vi "K2182A_Manage_Monitor.vi"(4 "System Monitor Variables (in)":T3, 5 "K2182A Cluster":T1 caption="Command (in)", 6 "Global Status (in)":T1, 7 "queue (in)":refnum<queue>) -> (0 "System Monitor Variables (out)":T3, 1 "Monitor (out)":T1)   [LabVIEW 2019]
uses:
  Global/Global Variables/System Monitor Cluster.ctl
  K2182A/K2812A_cluster.ctl
  Equipment/Keithley 622x/Configure/2182 -A/Low Level/Typedefs/KE2182 -- Voltage Ranges.ctl
  Equipment/Keithley 622x/Keithley 622x.lvlib
panel:
  # "K 2182A"
  # "K 2182A"
  # "K 2182A"
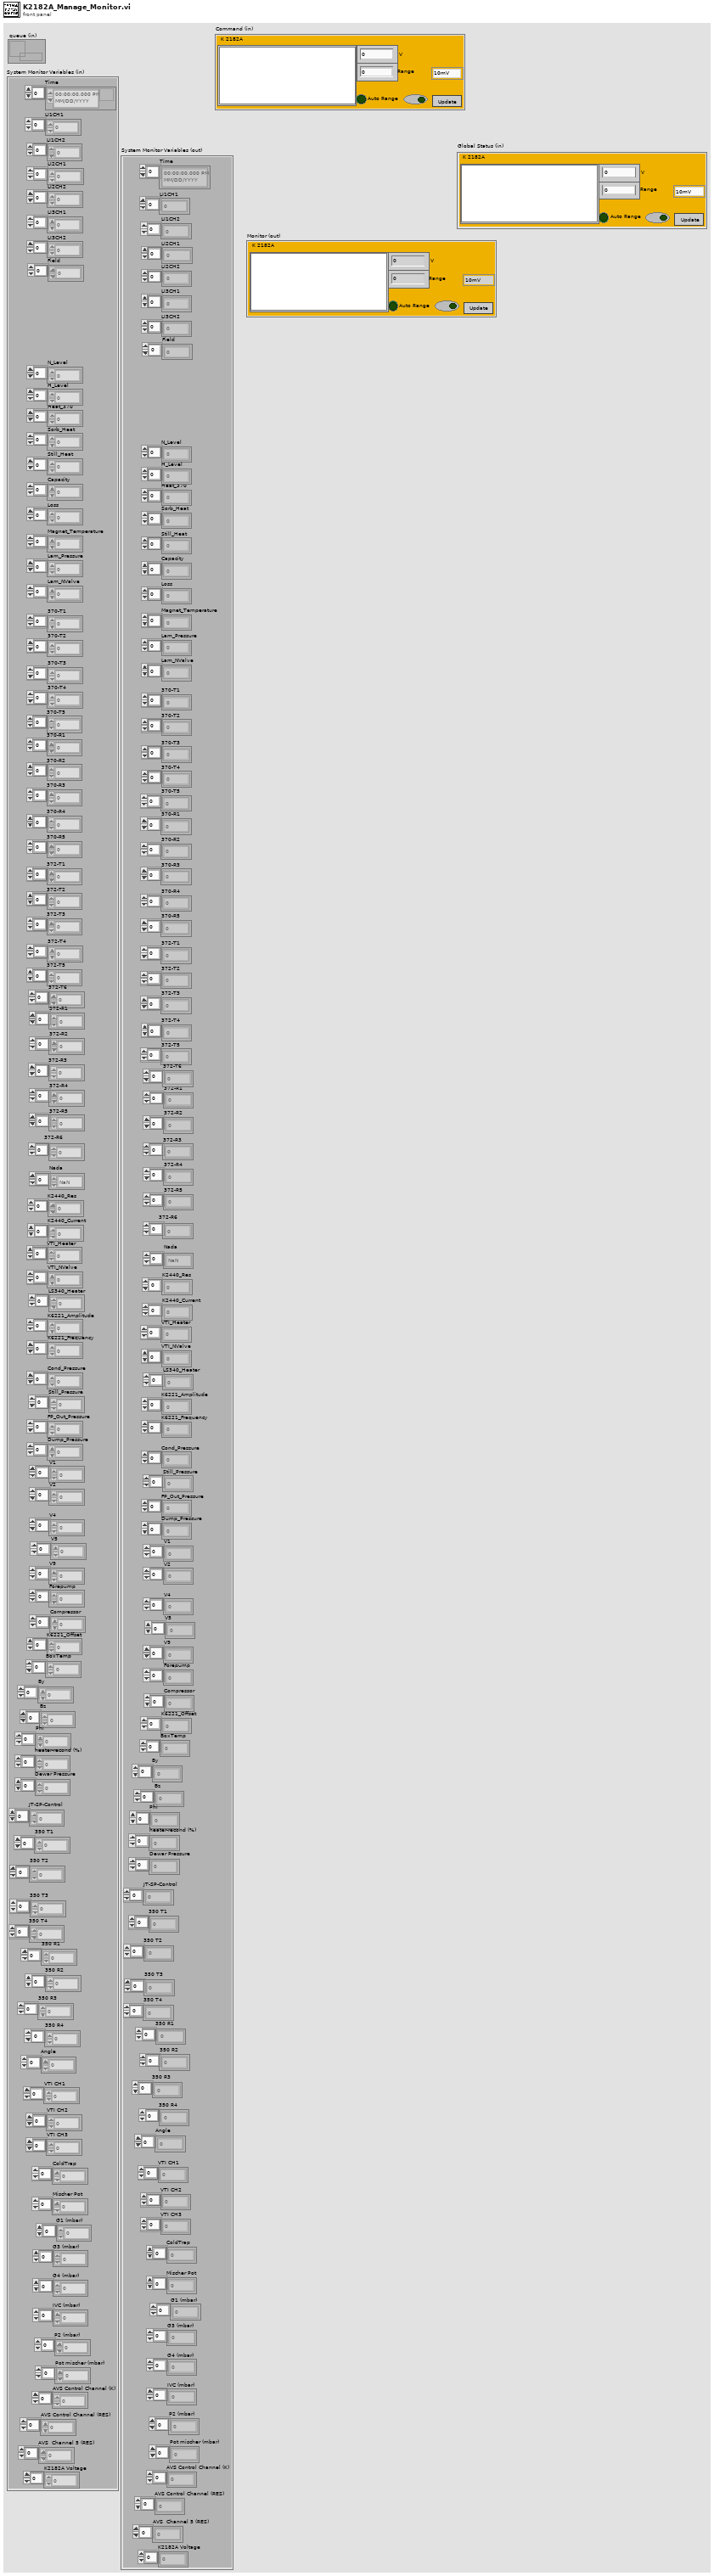
[diagram p1: front panel]
types:
  T1 = typedef "K2812A_cluster.ctl" = cluster{"Plot Window":dbl[][], "Range":dbl, "Update":bool, "Range selector":T2, "Auto Range":bool, "V":dbl, "Auto Range set":bool}
  T2 = typedef "Keithley 622x.lvlib/KE2182 -- Voltage Ranges.ctl" = enum16{"10mV", "100mV", "1V", "10V", "100V"}
  T3 = typedef "System Monitor Cluster.ctl" = cluster{"Time":timestamp[], "LI1CH1":dbl[], "LI1CH2":dbl[], "LI2CH1":dbl[], "LI2CH2":dbl[], "LI3CH1":dbl[], "LI3CH2":dbl[], "Field":dbl[], "N_Level":dbl[], "H_Level":dbl[], "Heat_370":dbl[], "Sorb_Heat":dbl[], "Still_Heat":dbl[], "Capacity":dbl[], "Loss":dbl[], "Magnet_Temperature":dbl[], "Lam_Pressure":dbl[], "Lam_NValve":dbl[], "370-T1":dbl[], "370-T2":dbl[], "370-T3":dbl[], "370-T4":dbl[], "370-T5":dbl[], "370-R1":dbl[], "370-R2":dbl[], "370-R3":dbl[], "370-R4":dbl[], "370-R5":dbl[], "372-T1":dbl[], "372-T2":dbl[], "372-T3":dbl[], "372-T4":dbl[], "372-T5":dbl[], "372-T6":dbl[], "372-R1":dbl[], "372-R2":dbl[], "372-R3":dbl[], "372-R4":dbl[], "372-R5":dbl[], "372-R6":dbl[], "Nada":dbl[], "K2440_Res":dbl[], "K2440_Current":dbl[], "VTI_Heater":dbl[], "VTI_NValve":dbl[], "LS340_Heater":dbl[], "K6221_Amplitude":dbl[], "K6221_Frequency":dbl[], "Cond_Pressure":dbl[], "Still_Pressure":dbl[], "FP_Out_Pressure":dbl[], "Dump_Pressure":dbl[], "V1":dbl[], "V2":dbl[], "V4":dbl[], "V5":dbl[], "V9":dbl[], "Forepump":dbl[], "Compressor":dbl[], "K6221_Offset":dbl[], "BoxTemp":dbl[], "By":dbl[], "Bz":dbl[], "Phi":dbl[], "heater-recond (%)":dbl[], "Dewar Pressure ":dbl[], "JT-SP-Control":dbl[], "350 T1":dbl[], "350 T2":dbl[], "350 T3":dbl[], "350 T4":dbl[], "350 R1":dbl[], "350 R2":dbl[], "350 R3":dbl[], "350 R4":dbl[], "Angle":dbl[], "VTI CH1":dbl[], "VTI CH2":dbl[], "VTI CH3":dbl[], "ColdTrap":dbl[], "Mischer Pot":dbl[], "G1 (mbar)":dbl[], "G3 (mbar) ":dbl[], "G4 (mbar)":dbl[], "IVC (mbar)":dbl[], "P2 (mbar) ":dbl[], "Pot mischer (mbar)":dbl[], "AVS Control Channel (K)":dbl[], "AVS Control Channel (RES)":dbl[], "AVS  Channel 5 (RES) ":dbl[], "K2182A Voltage":dbl[]}
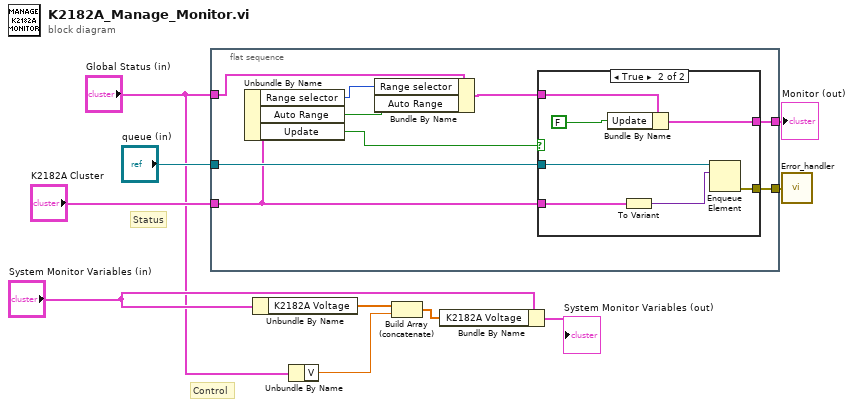
[diagram p0: block diagram]
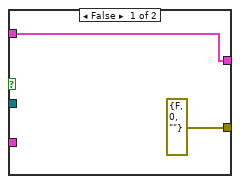
[diagram p2: hidden frame]
diagram:
  # "Status"
  # "Control"
  n1 = flat-sequence {
    tunnel: "queue (in)" -> [w19]
    tunnel: "K2182A Cluster" -> [w17]
    tunnel: [w18] -> w2
    tunnel: "Global Status (in)" -> [w14]
    tunnel: [w15] -> w1
    frame #0 {
      n2 = Unbundle By Name(w17) -> ("Range selector"=w12:T2, "Auto Range"=w11:bool, "Update"=w16:bool)
      n3 = Bundle By Name(cluster=w14, "Range selector"=w12, "Auto Range"=w11) -> (w13:T1)
      n4 = case shown="True" w16 {
        tunnel: w19 -> [_ w28]
        tunnel: w17 -> [_ w25]
        tunnel: [w20 w26] -> w18
        tunnel: w13 -> [w20 w24]
        tunnel: [errorcluster {"status"=FALSE, "code"=0, "source"=""} ("error constant") w23] -> w15
        frame False {
        }
        frame True {
          n5 = Bundle By Name(cluster=w24, "Update"=FALSE) -> (w26:T1)
          n6 = To Variant(anything=w25) -> (Variant=w27:variant)
          n7 = Enqueue Element(queue=w28, element=w27) -> (error out=w23:errorcluster)  [unwired: 2 in, 2 out]
        }
      }
    }
  }
  n8 = Unbundle By Name("System Monitor Variables (in)") -> ("K2182A Voltage"=w6:dbl[])
  n9 = Unbundle By Name("Global Status (in)") -> ("V"=w7:dbl)
  n10 = Build Array (concatenate)(w6, w7) -> (w5:dbl[])
  n11 = Bundle By Name(cluster="System Monitor Variables (in)", "K2182A Voltage"=w5) -> (→"System Monitor Variables (out)":T3)
  n12 = call "Error_handler.vi"("error constant"=w1) -> ()
  "Monitor (out)" <- w2
